vi "sub Console Append.vi"(4 "Console Ref":refnum<vi>, 5 "error in":errorcluster, 7 "String":string, 8 "VISA name":refnum<visa-resource-name>) -> (0 "error out":errorcluster, 1 "Console Out":refnum<vi>, 3 "VISA out":refnum<visa-resource-name>)   [LabVIEW 2025]
doc: "Used to append a string to the Command Logging text box. Inputs a reference to the text box and the string to append."
panel:
  # "GENESYS Power Supply\n Write Text to Console"
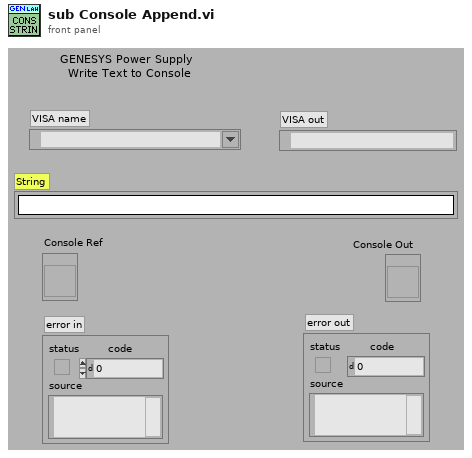
[diagram p1: front panel]
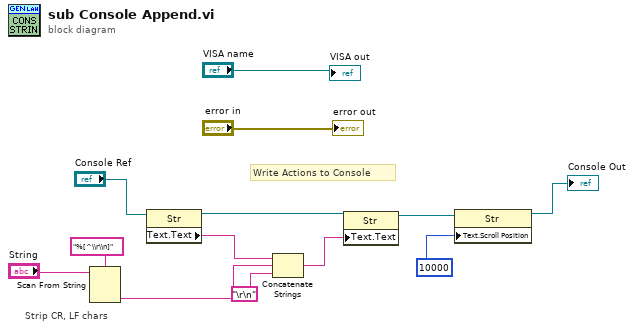
[diagram p0: block diagram]
diagram:
  # "Strip CR, LF chars"
  # "Write Actions to Console"
  n1 = Scan From String(format string="%[^\\r\\n]", input string="String") -> (output 1=w1:string)  [unwired: 3 in, 3 out]
  n2 = property class="Str"(reference="Console Ref") -> (reference out=w8:refnum<vi>, "Text.Text"=w9:string)  [unwired: 1 in, 1 out]
  n3 = Concatenate Strings(w9, w1, "\r\n") -> (w7:string)
  n4 = property class="Str"(reference=w8, "Text.Text"=w7) -> (reference out=w6:refnum<vi>)  [unwired: 1 in, 1 out]
  n5 = property class="Str"(reference=w6, "Text.Scroll Position"=u32 10000) -> (reference out=→"Console Out":refnum<vi>)  [unwired: 1 in, 1 out]
  "error out" <- "error in"
  "VISA out" <- "VISA name"
